vi "Read Lockin Processor Configuration.vi"(8 "error in (no error)":errorcluster, 11 "Lockin Processor in":refnum<class "Lockin Processor.lvclass">) -> (0 "error out":errorcluster, 2 "Configuration":T1={"Time constant"=0.0, "Phase"=0.0, "Signal channels"=[], "Group"="p", "X channel"="", "Live update"=TRUE} {"Phase" scale=-180.0..180.0; "Time constant" min=1e-06 max=1.0 scale=1e-06..0.01 scale format="%#_6p"}, 3 "Lockin Processor out":refnum<class "Lockin Processor.lvclass">)   [LabVIEW 2015, in "Lockin Processor.lvclass"]
uses:
  Lockin Processor.lvclass
  Lockin Processor Configuration.ctl
  Measure_core/Measure Object/Measure Object.lvclass/Measure Object.ctl
  Measure_core/Measure Object/Read Configuration.vi
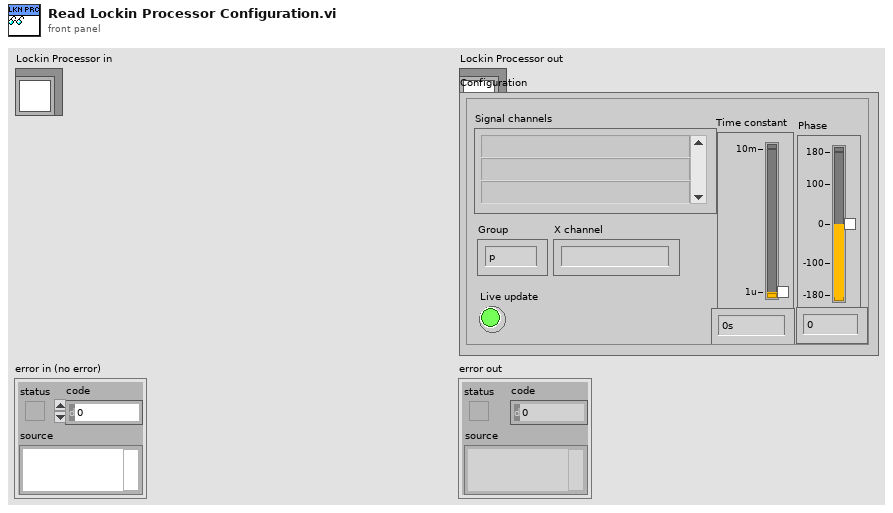
[diagram p1: front panel]
types:
  T1 = typedef "Lockin Processor Configuration.ctl" = cluster{"Time constant":dbl, "Phase":dbl, "Signal channels":string[], "Group":string, "X channel":string, "Live update":bool}
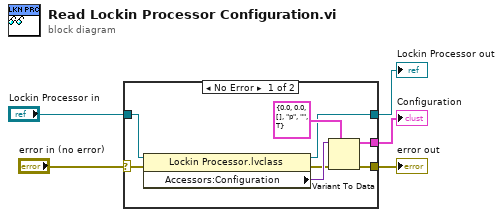
[diagram p0: block diagram]
diagram:
  n1 = case shown="No Error" "error in (no error)" {
    selector: "error in (no error)" -> [w6 w14]
    tunnel: [w12 w14] -> w4
    tunnel: [w10 w15] -> w2
    tunnel: "Lockin Processor in" -> [w13 w15]
    tunnel: [w8 _] -> w1
    frame No Error {
      n2 = property class="Lockin Processor.lvclass"(reference=w13, error in=w6) -> (reference out=w10:refnum<class "Lockin Processor.lvclass">, error out=w7:errorcluster, "Accessors:Configuration"=w9:variant)
      n3 = Variant To Data(error in=w7, type=T1 {"Time constant"=0.0, "Phase"=0.0, "Signal channels"=[], "Group"="p", "X channel"="", "Live update"=TRUE} ("Configuration"), Variant=w9) -> (data=w8:T1, error out=w12:errorcluster)
    }
    frame Error {
    }
  }
  "error out" <- w4
  "Lockin Processor out" <- w2
  "Configuration" <- w1
